vi "main.vi"() -> ()   [LabVIEW 2015, in "lv-recipe-machine.lvlib" / "example_02.lvlib"]
uses:
  example_02.lvlib
  _controls/customer.ctl
  _controls/tab_control.ctl
  public/_controls/mode.ctl
  public/_controls/automatic_state.ctl
  public/_controls/configuration.ctl
  _controls/fg_command.ctl
  lv-recipe-machine.lvlib
panel:
  in  "refresh_rate_ms":i32=-1
  out "step_elapsed_time":dbl format="%<%H:%M:%S>t"
  out "recipe_elapsed_time":dbl format="%<%H:%M:%S>t"
  out "step":string
  out "data":variant
  out "automatic_state":T1
  out "mode":T2
  in  "begin":bool
  out "error":errorcluster
  in  "exit":bool
  in  "next":bool
  in  "previous":bool
  in  "submit":bool
  out "tab_control":T3=enum."begin"
  in  "first_name":string
  in  "last_name":string
  in  "address_1":string
  in  "address_2":string
  in  "city":string
  in  "state":string
  in  "zip_code":string
  out "customer":T4
  # "Click submit to finish"
  # "Click begin to start"
  # "Click begin to start"
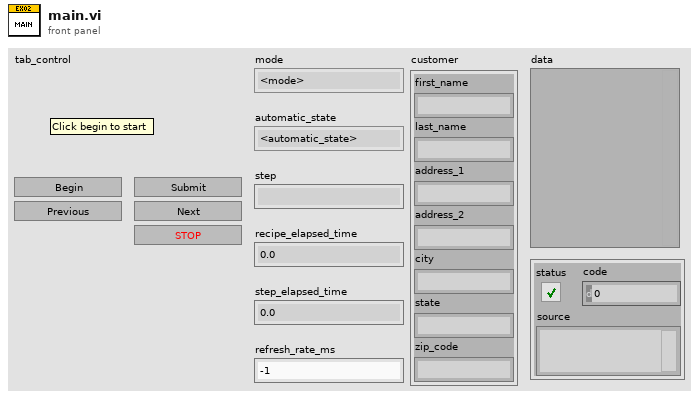
[diagram p1: front panel]
types:
  T1 = typedef "lv-recipe-machine.lvlib/automatic_state.ctl" = enum16{"<automatic_state>", "failed", "idle", "running", "paused", "stopped", "<null>"}
  T2 = typedef "lv-recipe-machine.lvlib/mode.ctl" = enum16{"<mode>", "manual", "automatic", "<null>"}
  T3 = typedef "lv-recipe-machine.lvlib/example_02.lvlib/tab_control.ctl" = enum32{"first_name", "last_name", "address", "city", "state", "zip_code", "submit", "begin"}
  T4 = typedef "lv-recipe-machine.lvlib/example_02.lvlib/customer.ctl" = cluster{"first_name":string, "last_name":string, "address_1":string, "address_2":string, "city":string, "state":string, "zip_code":string}
  T5 = typedef "lv-recipe-machine.lvlib/example_02.lvlib/fg_command.ctl" = enum16{"<fg_command>", "initialize", "read", "write", "shutdown"}
  T6 = typedef "lv-recipe-machine.lvlib/configuration.ctl" = cluster{"change_in_timeout_ms":i32}
  T7 = cluster{"change_out":refnum<event-registration>, "status_event_registration":refnum<event-registration>}
  T8 = typedef "lv-recipe-machine.lvlib/recipe_step.ctl" = cluster{"step":string, "data":variant}
  T9 = typedef "lv-recipe-machine.lvlib/status.ctl" = cluster{"mode":T2, "manual_state":T10, "automatic_state":T1, "automatic_data":variant, "step":string, "recipe_elapsed_time":dbl, "step_elapsed_time":dbl, "recipe_error":errorcluster}
  T10 = typedef "lv-recipe-machine.lvlib/manual_state.ctl" = enum16{"<manual_state>", "failed", "action", "running", "idle", "<null>"}
  T11 = typedef "example_02.lvlib/tab_control.ctl" = enum32{"first_name", "last_name", "address", "city", "state", "zip_code", "submit", "begin"}
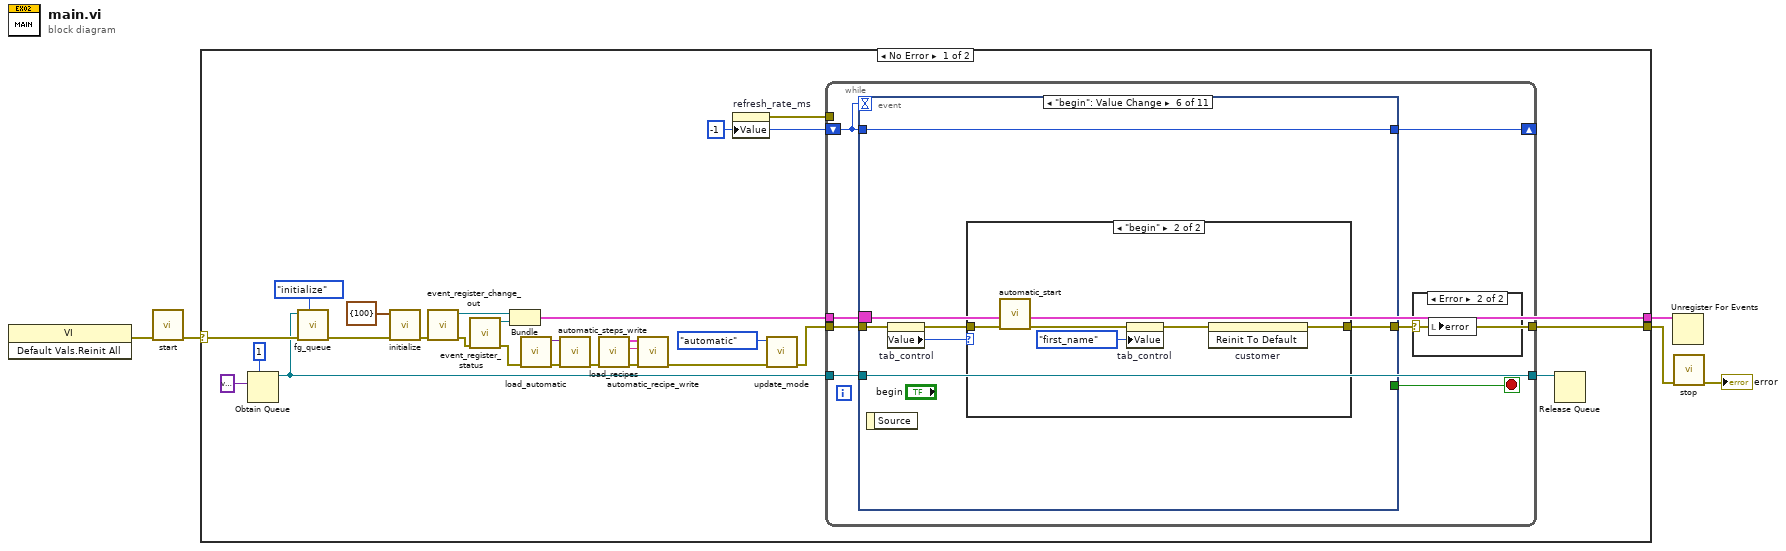
[diagram p0: block diagram]
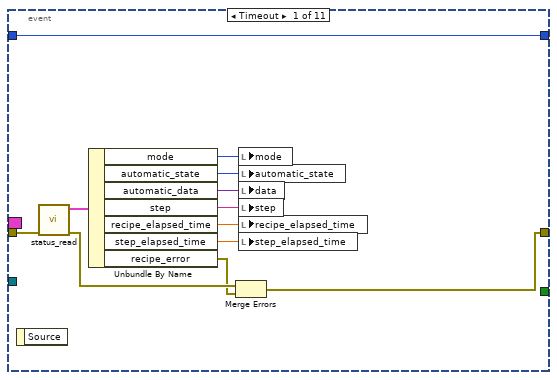
[diagram p2: hidden frame]
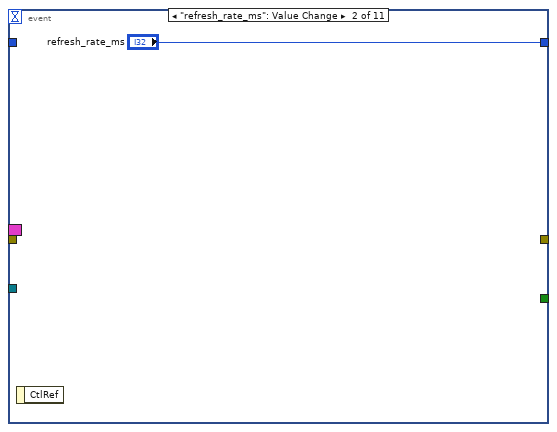
[diagram p3: hidden frame]
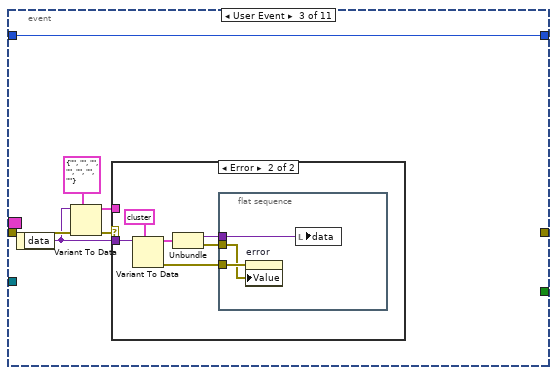
[diagram p4: hidden frame]
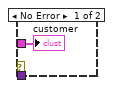
[diagram p5: hidden frame]
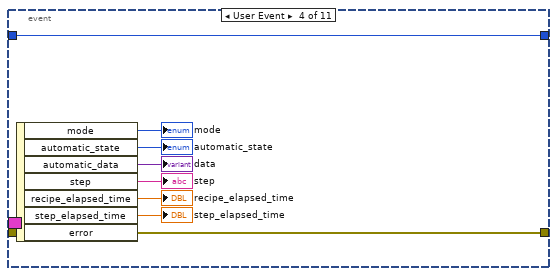
[diagram p6: hidden frame]
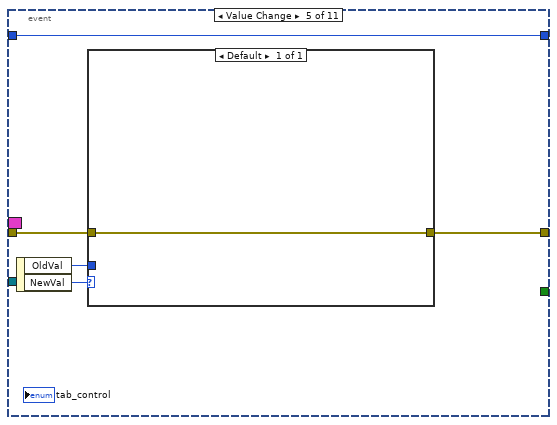
[diagram p7: hidden frame]
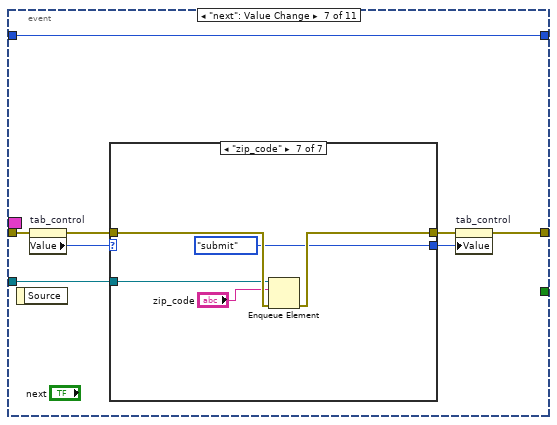
[diagram p9: hidden frame]
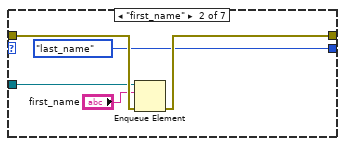
[diagram p11: hidden frame]
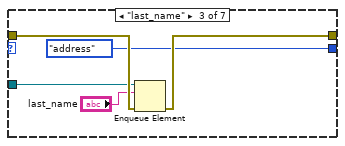
[diagram p12: hidden frame]
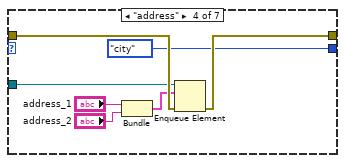
[diagram p13: hidden frame]
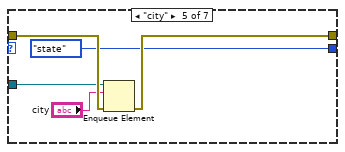
[diagram p14: hidden frame]
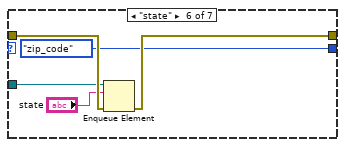
[diagram p15: hidden frame]
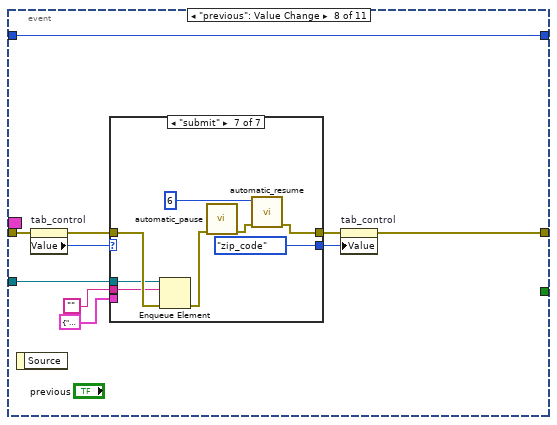
[diagram p16: hidden frame]
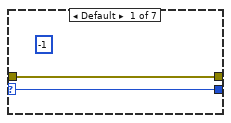
[diagram p17: hidden frame]
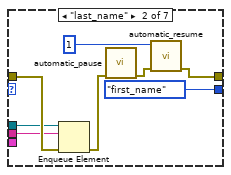
[diagram p18: hidden frame]
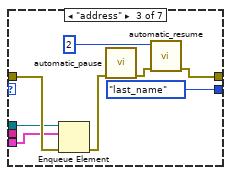
[diagram p19: hidden frame]
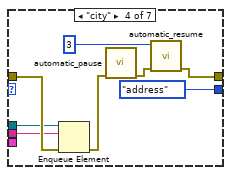
[diagram p20: hidden frame]
diagram:
  n1 = invoke class="VI" method="Default Vals.Reinit All"() -> (error out=w5:errorcluster)  [unwired: 3 in, 2 out]
  n2 = call "start.vi"("error in (no error)"=w5) -> ("error out"=w2:errorcluster)  [unwired: 10 in]
  n3 = case shown="No Error" w2 {
    selector: w2 -> [w31 w215]
    tunnel: [w24 w215] -> w4
    tunnel: [w23 _] -> w1
    frame No Error {
      w10 = -1
      n4 = Obtain Queue(max queue size (-1, unlimited)=1, element data type=variant) -> (queue out=w11:refnum<queue>)  [unwired: 3 in, 2 out]
      n5 = call "fg_queue.vi"("command"=fg_command."initialize", "error in (no error)"=w31, "queue in"=w11) -> ("error out"=w16:errorcluster)  [unwired: 7 in, 1 out]
      n6 = call "initialize.vi"("error in (no error)"=w16, "configuration"=T6 {"change_in_timeout_ms"=100}) -> ("error out"=w17:errorcluster)  [unwired: 9 in]
      n7 = call "event_register_change_out.vi"("error in (no error)"=w17) -> ("error out"=w25:errorcluster, "change_out"=w27:refnum<event-registration>)  [unwired: 9 in]
      n8 = call "event_register_status.vi"("error in (no error)"=w25) -> ("error out"=w8:errorcluster, "status_event_registration"=w26:refnum<event-registration>)  [unwired: 9 in]
      n9 = Bundle("change_out"=w27, "status_event_registration"=w26) -> (w23:T7)  [unwired: 1 in]
      n10 = call "load_automatic.vi"("error in (no error)"=w8) -> ("error out"=w29:errorcluster, "automatic_steps out"=w28:variant)  [unwired: 8 in, 1 out]
      n11 = call "automatic_steps_write.vi"("error in (no error)"=w29, "automatic_steps"=w28) -> ("error out"=w19:errorcluster)  [unwired: 8 in, 1 out]
      n12 = call "load_recipes.vi"("error in (no error)"=w19) -> ("error out"=w20:errorcluster, "transition []"=w21:string, "recipe []"=w22:T8[])  [unwired: 8 in]
      n13 = call "automatic_recipe_write.vi"("error in (no error)"=w20, "transition"=w21, "recipe []"=w22) -> ("error out"=w7:errorcluster)  [unwired: 8 in]
      n14 = property on="refresh_rate_ms" class="DigNum (strict)"("Value"=w10) -> (error out=w9:errorcluster)  [unwired: 2 in, 1 out]
      n15 = call "update_mode.vi"("error in (no error)"=w7, "mode"=mode."automatic") -> ("error out"=w6:errorcluster)  [unwired: 9 in]
      n16 = while {
        tunnel: w6 -> [w37]
        tunnel: [w36] -> w24
        tunnel: w23 -> [w35]
        shift-right: [w34] -> _
        shift-left: w10 -> [w33]
        tunnel: w11 -> [w32]
        tunnel: [w32] -> w13
        tunnel: w9 -> [_]
        stop <- w38 stop-if-true
        n17 = event shown="[5] \"begin\": Value Change" {
          selector: w35 -> [_ _ _ _ _ _ _ _ _ _ _]
          dyn-events: _ -> [_ _ _ _ _ _ _ _ _ _ _]
          timeout: w33 -> [_ _ _ _ _ _ _ _ _ _ _]
          tunnel: [_ _ _ _ _ _ _ _ _ w210 TRUE] -> w38
          tunnel: w37 -> [w49 _ w56 _ w77 w84 w99 w143 w200 _ w211]
          tunnel: [w45 _ _ w68 w76 w85 w96 w142 w199 _ w211] -> w36
          tunnel: w33 -> [w50 _ w57 w75 w80 w86 w100 w144 w201 w209 w212]
          tunnel: [w50 "refresh_rate_ms" w57 w75 w80 w86 w100 w144 w201 w209 w212] -> w34
          tunnel: w32 -> [_ _ _ _ _ _ w94 w138 w196 _ _]
          event Timeout {
            n18 = event-data() -> ()  [unwired: 1 in, 1 out]
            n19 = call "status_read.vi"("error in (no error)"=w49) -> ("error out"=w47:errorcluster, "status"=w48:T9)  [unwired: 9 in]
            n20 = Unbundle By Name(w48) -> ("mode"=w44:T2, "automatic_state"=w43:T1, "automatic_data"=w42:variant, "step"=w41:string, "recipe_elapsed_time"=w40:dbl, "step_elapsed_time"=w39:dbl, "recipe_error"=w46:errorcluster)
            n21 = Merge Errors(w47, w46) -> (w45:errorcluster)
            n22 = local write "mode"(w44) -> ()
            n23 = local write "automatic_state"(w43) -> ()
            n24 = local write "data"(w42) -> ()
            n25 = local write "step"(w41) -> ()
            n26 = local write "recipe_elapsed_time"(w40) -> ()
            n27 = local write "step_elapsed_time"(w39) -> ()
          }
          event "refresh_rate_ms": Value Change {
            n28 = event-data() -> ()  [unwired: 1 in, 1 out]
          }
          event User Event {
            n29 = event-data() -> ("data"=w52:variant)  [unwired: 1 in]
            n30 = Variant To Data(error in=w56, type=T4 {"first_name"="", "last_name"="", "address_1"="", "address_2"="", "city"="", "state"="", "zip_code"=""} ("customer"), Variant=w52) -> (data=w55:T4, error out=w53:errorcluster)
            n31 = case shown="Error" w53 {
              tunnel: w55 -> [w58 _]
              tunnel: w52 -> [_ w59]
              frame No Error {
                "customer" <- w58
              }
              frame Error {
                n32 = Variant To Data(type=cluster{variant, "error constant":errorcluster} {variant, "error constant"={"status"=FALSE, "code"=0, "source"=""}}, Variant=w59) -> (data=w60:cluster{variant, "error constant":errorcluster}, error out=w64:errorcluster)  [unwired: 1 in]
                n33 = Unbundle(w60) -> (w62:variant, "error constant"=w63:errorcluster)
                n34 = flat-sequence {
                  tunnel: w62 -> [w65]
                  tunnel: w63 -> [w66]
                  tunnel: w64 -> [w67]
                  frame #0 {
                    n35 = property on="error" class="Clust (strict)"(error in=w67, "Value"=w66) -> ()  [unwired: 1 in, 2 out]
                    n36 = local write "data"(w65) -> ()
                  }
                }
              }
            }
          }
          event User Event {
            n37 = event-data() -> ("mode"=→"mode":T2, "automatic_state"=→"automatic_state":T1, "automatic_data"=→"data":variant, "step"=→"step":string, "recipe_elapsed_time"=→"recipe_elapsed_time":dbl, "step_elapsed_time"=→"step_elapsed_time":dbl, "error"=w68:errorcluster)  [unwired: 1 in]
          }
          event Value Change {
            n38 = event-data() -> ("OldVal"=w78:T3, "NewVal"=w79:T3)  [unwired: 1 in]
            n39 = case shown="Default" w79 {
              tunnel: w78 -> [_]
              tunnel: w77 -> [w81]
              tunnel: [w81] -> w76
              frame Default {
              }
            }
          }
          event "begin": Value Change {
            n40 = event-data() -> ()  [unwired: 1 in, 1 out]
            n41 = property on="tab_control" class="TabCtl (strict)"(error in=w84) -> (error out=w83:errorcluster, "Value"=w82:T11)  [unwired: 1 in, 1 out]
            n42 = case shown="\"begin\"" w82 {
              tunnel: [w87 w88] -> w85
              tunnel: w83 -> [w87 w90]
              frame Default {
              }
              frame "begin" {
                n43 = call "automatic_start.vi"("error in (no error)"=w90) -> ("error out"=w92:errorcluster)  [unwired: 10 in]
                n44 = property on="tab_control" class="TabCtl (strict)"(error in=w92, "Value"=tab_control."first_name" ("tab_control")) -> (error out=w89:errorcluster)  [unwired: 1 in, 1 out]
                n45 = invoke on="customer" class="Clust (strict)" method="Reinit To Default"(error in=w89) -> (error out=w88:errorcluster)  [unwired: 2 in, 2 out]
              }
            }
          }
          event "next": Value Change {
            n46 = event-data() -> ()  [unwired: 1 in, 1 out]
            n47 = property on="tab_control" class="TabCtl (strict)"(error in=w99) -> (error out=w97:errorcluster, "Value"=w98:T11)  [unwired: 1 in, 1 out]
            n48 = case shown="\"zip_code\"" w98 {
              selector: w98 -> [w101 _ _ _ _ _ _]
              tunnel: w97 -> [w102 w107 w112 w119 w124 w129 w134]
              tunnel: [w102 w106 w111 w118 w123 w128 w133] -> w93
              tunnel: [w101 tab_control."last_name" ("tab_control") tab_control."address" ("tab_control") tab_control."city" ("tab_control") tab_control."state" ("tab_control") tab_control."zip_code" ("tab_control") tab_control."submit" ("tab_control")] -> w95
              tunnel: w94 -> [_ w104 w109 w116 w121 w126 w131]
              frame Default {
              }
              frame "first_name" {
                n49 = Enqueue Element(queue=w104, element="first_name", error in (no error)=w107) -> (error out=w106:errorcluster)  [unwired: 1 in, 2 out]
              }
              frame "last_name" {
                n50 = Enqueue Element(queue=w109, element="last_name", error in (no error)=w112) -> (error out=w111:errorcluster)  [unwired: 1 in, 2 out]
              }
              frame "address" {
                n51 = Bundle("address_1"="address_1", "address_2"="address_2") -> (w115:cluster{"address_1":string, "address_2":string})  [unwired: 1 in]
                n52 = Enqueue Element(queue=w116, element=w115, error in (no error)=w119) -> (error out=w118:errorcluster)  [unwired: 1 in, 2 out]
              }
              frame "city" {
                n53 = Enqueue Element(queue=w121, element="city", error in (no error)=w124) -> (error out=w123:errorcluster)  [unwired: 1 in, 2 out]
              }
              frame "state" {
                n54 = Enqueue Element(queue=w126, element="state", error in (no error)=w129) -> (error out=w128:errorcluster)  [unwired: 1 in, 2 out]
              }
              frame "zip_code" {
                n55 = Enqueue Element(queue=w131, element="zip_code", error in (no error)=w134) -> (error out=w133:errorcluster)  [unwired: 1 in, 2 out]
              }
            }
            n56 = property on="tab_control" class="TabCtl (strict)"(error in=w93, "Value"=w95) -> (error out=w96:errorcluster)  [unwired: 1 in, 1 out]
          }
          event "previous": Value Change {
            n57 = event-data() -> ()  [unwired: 1 in, 1 out]
            n58 = property on="tab_control" class="TabCtl (strict)"(error in=w143) -> (error out=w140:errorcluster, "Value"=w141:T11)  [unwired: 1 in, 1 out]
            n59 = case shown="\"submit\"" w141 {
              selector: w141 -> [w145 _ _ _ _ _ _]
              tunnel: w140 -> [w146 w154 w162 w170 w178 w186 w194]
              tunnel: [w145 tab_control."first_name" ("tab_control") tab_control."last_name" ("tab_control") tab_control."address" ("tab_control") tab_control."city" ("tab_control") tab_control."state" ("tab_control") tab_control."zip_code" ("tab_control")] -> w139
              tunnel: [w146 w147 w156 w164 w172 w180 w188] -> w135
              tunnel: "" -> [_ w152 _ w163 w171 w179 w187]
              tunnel: w138 -> [_ w151 w160 w168 w176 w184 w192]
              tunnel: cluster{string, string} {"", ""} -> [_ _ w155 _ _ _ _]
              frame Default {
                (unwired) -1
              }
              frame "last_name" {
                n60 = Enqueue Element(queue=w151, element=w152, error in (no error)=w154) -> (error out=w148:errorcluster)  [unwired: 1 in, 2 out]
                n61 = call "automatic_pause.vi"("error in (no error)"=w148) -> ("error out"=w149:errorcluster)  [unwired: 10 in]
                n62 = call "automatic_resume.vi"("error in (no error)"=w149, "index"=1) -> ("error out"=w147:errorcluster)  [unwired: 9 in]
              }
              frame "address" {
                n63 = Enqueue Element(queue=w160, element=w155, error in (no error)=w162) -> (error out=w157:errorcluster)  [unwired: 1 in, 2 out]
                n64 = call "automatic_pause.vi"("error in (no error)"=w157) -> ("error out"=w158:errorcluster)  [unwired: 10 in]
                n65 = call "automatic_resume.vi"("error in (no error)"=w158, "index"=2) -> ("error out"=w156:errorcluster)  [unwired: 9 in]
              }
              frame "city" {
                n66 = Enqueue Element(queue=w168, element=w163, error in (no error)=w170) -> (error out=w165:errorcluster)  [unwired: 1 in, 2 out]
                n67 = call "automatic_pause.vi"("error in (no error)"=w165) -> ("error out"=w166:errorcluster)  [unwired: 10 in]
                n68 = call "automatic_resume.vi"("error in (no error)"=w166, "index"=3) -> ("error out"=w164:errorcluster)  [unwired: 9 in]
              }
              frame "state" {
                n69 = Enqueue Element(queue=w176, element=w171, error in (no error)=w178) -> (error out=w173:errorcluster)  [unwired: 1 in, 2 out]
                n70 = call "automatic_pause.vi"("error in (no error)"=w173) -> ("error out"=w174:errorcluster)  [unwired: 10 in]
                n71 = call "automatic_resume.vi"("error in (no error)"=w174, "index"=4) -> ("error out"=w172:errorcluster)  [unwired: 9 in]
              }
              frame "zip_code" {
                n72 = Enqueue Element(queue=w184, element=w179, error in (no error)=w186) -> (error out=w181:errorcluster)  [unwired: 1 in, 2 out]
                n73 = call "automatic_pause.vi"("error in (no error)"=w181) -> ("error out"=w182:errorcluster)  [unwired: 10 in]
                n74 = call "automatic_resume.vi"("error in (no error)"=w182, "index"=5) -> ("error out"=w180:errorcluster)  [unwired: 9 in]
              }
              frame "submit" {
                n75 = Enqueue Element(queue=w192, element=w187, error in (no error)=w194) -> (error out=w189:errorcluster)  [unwired: 1 in, 2 out]
                n76 = call "automatic_pause.vi"("error in (no error)"=w189) -> ("error out"=w190:errorcluster)  [unwired: 10 in]
                n77 = call "automatic_resume.vi"("error in (no error)"=w190, "index"=6) -> ("error out"=w188:errorcluster)  [unwired: 9 in]
              }
            }
            n78 = property on="tab_control" class="TabCtl (strict)"(error in=w135, "Value"=w139) -> (error out=w142:errorcluster)  [unwired: 1 in, 1 out]
          }
          event "submit": Value Change {
            n79 = event-data() -> ()  [unwired: 1 in, 1 out]
            n80 = property on="tab_control" class="TabCtl (strict)"(error in=w200) -> (error out=w198:errorcluster, "Value"=w197:T11)  [unwired: 1 in, 1 out]
            n81 = case shown="\"submit\"" w197 {
              tunnel: [w202 w207] -> w199
              tunnel: w198 -> [w202 w208]
              tunnel: variant -> [_ w205]
              tunnel: w196 -> [_ w203]
              frame Default {
              }
              frame "submit" {
                n82 = Enqueue Element(queue=w203, element=w205, error in (no error)=w208) -> (error out=w204:errorcluster)  [unwired: 1 in, 2 out]
                n83 = property on="tab_control" class="TabCtl (strict)"(error in=w204, "Value"=tab_control."begin" ("tab_control")) -> (error out=w207:errorcluster)  [unwired: 1 in, 1 out]
              }
            }
          }
          event Panel Close? {
            w210 = TRUE
            n84 = event-data() -> ()  [unwired: 1 in, 1 out]
            n85 = event-data("Discard?"=w210) -> ()  [unwired: 1 in, 1 out]
          }
          event "exit": Value Change {
            n86 = event-data() -> ()  [unwired: 1 in, 1 out]
          }
        }
        n87 = case shown="Error" w36 {
          selector: w36 -> [_ w214]
          frame No Error {
          }
          frame Error {
            n88 = local write "error"(w214) -> ()
          }
        }
      }
      n89 = Release Queue(queue=w13) -> ()  [unwired: 2 in, 3 out]
    }
    frame Error {
    }
  }
  n90 = Unregister For Events(event registration refnum=w1) -> ()  [unwired: 1 in, 1 out]
  n91 = call "stop.vi"("error in (no error)"=w4) -> ("error out"=→"error":errorcluster)  [unwired: 10 in]
